vi "search.vi"(8 "xy":dbl[][](array[numeric]), 10 "x":dbl, 11 "y":dbl) -> (0 "Numeric":dbl)   [LabVIEW 2013]
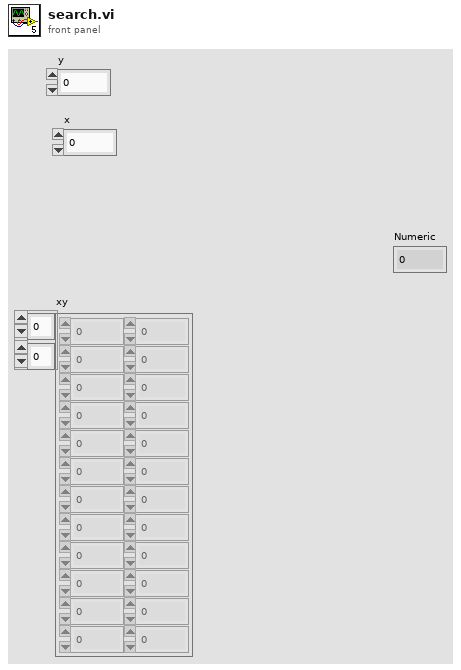
[diagram p1: front panel]
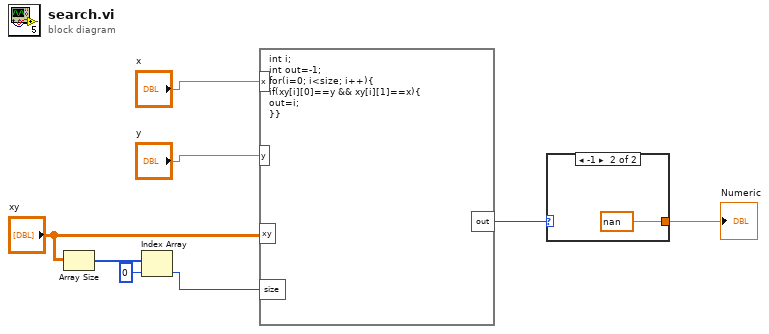
[diagram p0: block diagram]
diagram:
  n1 = Array Size(array="xy") -> (size(s)=w5:i32[])
  n2 = Index Array(array=w5, index=0) -> (element=w3:i32)
  n3 = formula code="int i;\nint out=-1;\nfor(i=0; i<size; i++){\nif(xy[i][0]==y && xy[i][1]==x){\nout=i;\n}}"("x"="x", "y"="y", "xy"="xy", "size"=w3) -> ("out"=w2:i32)
  n4 = case shown="-1" w2 {
    selector: w2 -> [w9 _]
    tunnel: [w9 nan] -> w1
    frame Default {
    }
    frame -1 {
    }
  }
  "Numeric" <- w1
